vi "Move Inc.vi"(6 "Axis":string, 8 "error in (no error)":errorcluster, 9 "Speed":dbl format="%#_13g", 10 "Distance":dbl format="%#_13g", 11 "Gantry In":refnum<k24>) -> (0 "error out":errorcluster, 3 "Gantry Out":refnum<k24>)   [LabVIEW 2018, in "A3200.lvclass"]
uses:
  A3200.lvclass
  C:/Program Files (x86)/Aerotech/A3200/LabVIEW/2010/Bin/Aerotech.A3200.dll
  Program Files (x86)/Aerotech/A3200/LabVIEW/2010/Bin/Aerotech.A3200.dll
  Drivers/Aerotech A3200/Aerotech.lvlib
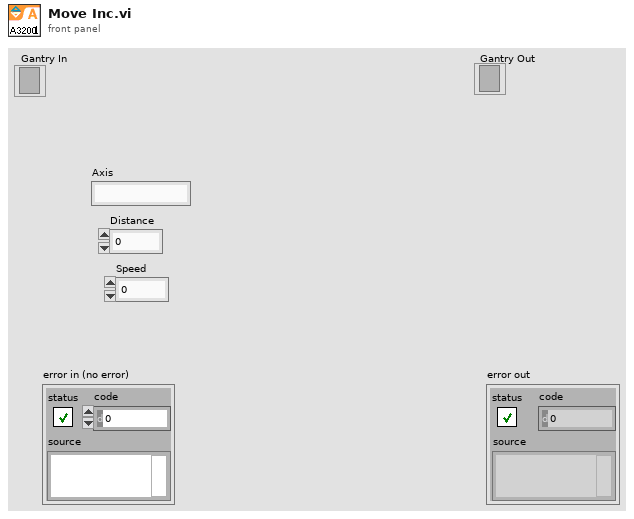
[diagram p1: front panel]
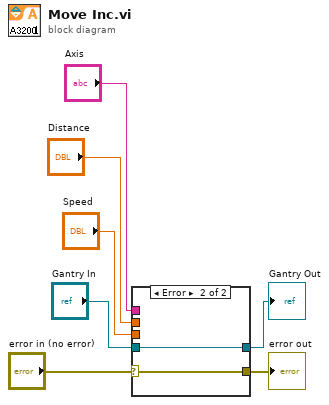
[diagram p0: block diagram]
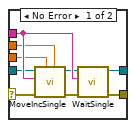
[diagram p2: hidden frame]
diagram:
  n1 = case shown="Error" "error in (no error)" {
    selector: "error in (no error)" -> [w12 w18]
    tunnel: [w10 w18] -> w6
    tunnel: "Axis" -> [w16 _]
    tunnel: "Speed" -> [w15 _]
    tunnel: "Distance" -> [w14 _]
    tunnel: "Gantry In" -> [w9 w17]
    tunnel: [w8 w17] -> w1
    frame No Error {
      n2 = call "MoveIncSingle.vi"("distance"=w14, "speed"=w15, "error in (no error)"=w12, "axis name"=w16, "controller in"=w9) -> ("error out"=w11:errorcluster, "controller out"=w13:refnum<k24>)  [unwired: 5 in]
      n3 = call "WaitSingle.vi"("error in (no error)"=w11, "axis name"=w16, "controller in"=w13) -> ("error out"=w10:errorcluster, "controller out"=w8:refnum<k24>)  [unwired: 6 in, 1 out]
    }
    frame Error {
    }
  }
  "error out" <- w6
  "Gantry Out" <- w1
